vi "CompareWaveformSizes.vi"(8 "error in (no error)":errorcluster, 11 "ClassIn":refnum<class "NiPxi6733.lvclass">) -> (0 "error out":errorcluster, 2 "WaveformSize":i32, 3 "ClassOut":refnum<class "NiPxi6733.lvclass">)   [LabVIEW 2014, in "FGenPlugins.lvlib" / "NiPxi6733.lvclass"]
uses:
  NiPxi6733.lvclass
  <vilib>/Utility/error.llb/Error Cluster From Error Code.vi
  <vilib>/ErrorRing/Error Ring.xnode
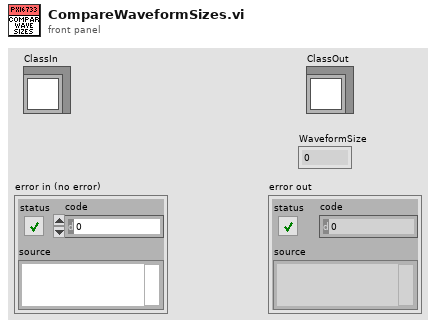
[diagram p1: front panel]
types:
  T1 = typedef "FGenPlugins.lvlib/NISTFGenPluginsBase.lvclass/ChannelParamElement.ctl" = cluster{"sName":string, "eOperateMode":u16, "bEnabled":bool, "eOutputMode":u16, "iIndex":i32, "iNameBufferSize":i32, "fGain":dbl}
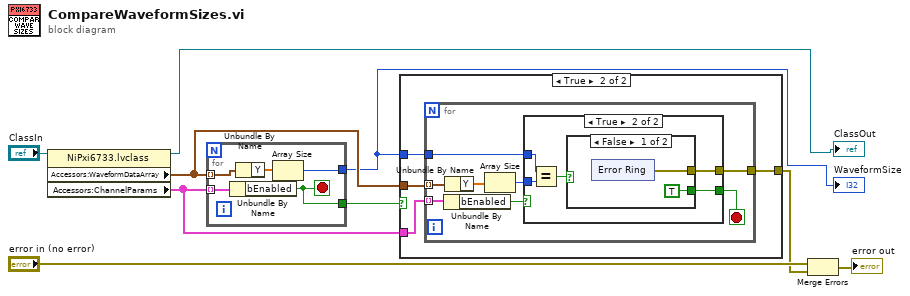
[diagram p0: block diagram]
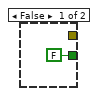
[diagram p3: hidden frame]
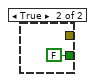
[diagram p4: hidden frame]
diagram:
  n1 = property class="NiPxi6733.lvclass"(reference="ClassIn") -> (reference out=→"ClassOut":refnum<class "NiPxi6733.lvclass">, "Accessors:WaveformDataArray"=w7:waveform(dbl)[], "Accessors:ChannelParams"=w5:T1[])  [unwired: 1 in, 1 out]
  n2 = for {
    tunnel: w5 -> [w14] mode=indexing
    tunnel: w7 -> [w13] mode=indexing
    tunnel: [w11] -> w1
    tunnel: [w10] -> w6
    stop <- w10 stop-if-true
    n3 = Unbundle By Name(w14) -> ("bEnabled"=w10:bool)
    n4 = Unbundle By Name(w13) -> ("Y"=w12:dbl[])
    n5 = Array Size(array=w12) -> (size(s)=w11:i32)
  }
  "WaveformSize" <- w1
  n6 = case shown="True" w6 {
    tunnel: w7 -> [_ w18]
    tunnel: w1 -> [_ w17]
    tunnel: w5 -> [_ w16]
    tunnel: [_ w15] -> w2
    frame False {
    }
    frame True {
      n7 = for {
        tunnel: w18 -> [w25] mode=indexing
        tunnel: w16 -> [w24] mode=indexing
        tunnel: w17 -> [w21]
        tunnel: [w19] -> w15
        stop <- w20 stop-if-true
        n8 = Unbundle By Name(w24) -> ("bEnabled"=w23:bool)
        n9 = Unbundle By Name(w25) -> ("Y"=w26:dbl[])
        n10 = Array Size(array=w26) -> (size(s)=w22:i32)
        n11 = case shown="True" w23 {
          tunnel: w22 -> [_ w32]
          tunnel: w21 -> [_ w31]
          tunnel: [FALSE w29] -> w20
          tunnel: [_ w28] -> w19
          frame False {
          }
          frame True {
            n12 = Equal?(x=w31, y=w32) -> (x = y?=w30:bool)
            n13 = case shown="False" w30 {
              tunnel: [TRUE FALSE] -> w29
              tunnel: [w33 _] -> w28
              frame False {
                n14 = xnode "Error Ring"() -> ("error out"=w33:errorcluster)
              }
              frame True {
              }
            }
          }
        }
      }
    }
  }
  n15 = Merge Errors("error in (no error)", w2) -> (→"error out":errorcluster)
